vi "Thev-Test Find Fq.vi"() -> ()   [LabVIEW 2015]
panel:
  in  "Path":path=path "D:/Data/FPL/Example.2/37.0mm.calib"
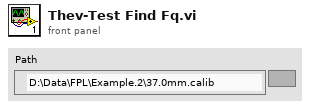
[diagram p1: front panel]
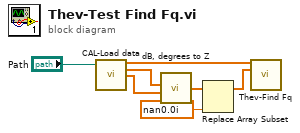
[diagram p0: block diagram]
diagram:
  n1 = call "CAL-Load data.vi"("user path"="Path") -> ("Frequency (Hz)"=w4:dbl[], "Mag"=w6:dbl[], "Phase"=w5:dbl[])  [unwired: 7 in, 5 out]
  n2 = call "dB, degrees to Z.vi"("Magnitude (dB)"=w6, "Phase (degrees)"=w5) -> ("Z"=w3:cdb[])  [unwired: 5 in]
  n3 = Replace Array Subset(array=w3, new element=cdb nan+0.0i ("new element/subarray")) -> (w2:cdb[])  [unwired: 1 in]
  n4 = call "Thev-Find Fq.vi"("Frequency (Hz)"=w4, "Px"=w2) -> ()  [unwired: 13 in, 1 out]
